vi "Swerve Goto.vi"(1 "Target Angle":dbl, 2 "Target Y":dbl, 3 "Target X":dbl, 4 "Max Speed":dbl) -> (0 "Done":bool)   [LabVIEW 2016, in "Apple script.lvlib"]
uses:
  Apple script.lvlib
  Robot Global Data.vi
  <vilib>/addons/control/pid/NI_PID_pid.lvlib
  <vilib>/addons/control/pid/pid.llb/PID (DBL).vi
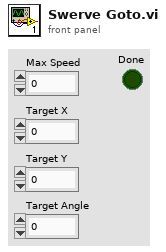
[diagram p1: front panel]
types:
  T1 = enum16{"Prepare to Rotate", "Rotate", "Prepare to Move", "Move", "Done"}
  T2 = cluster{"proportional gain (Kc)":dbl, "integral time (Ti, min)":dbl, "derivative time (Td, min)":dbl}
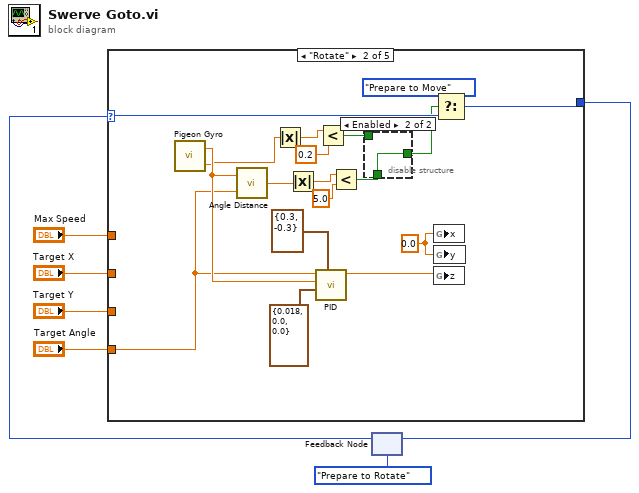
[diagram p0: block diagram]
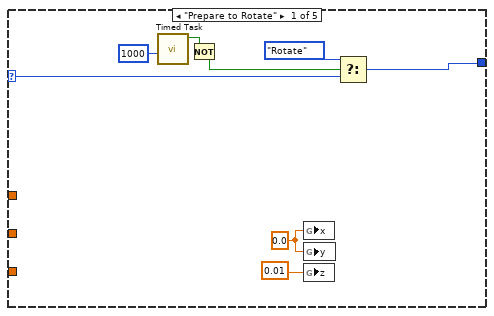
[diagram p2: hidden frame]
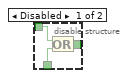
[diagram p3: hidden frame]
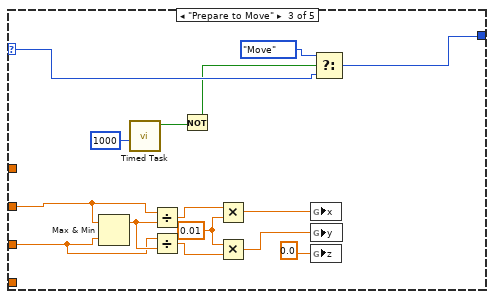
[diagram p4: hidden frame]
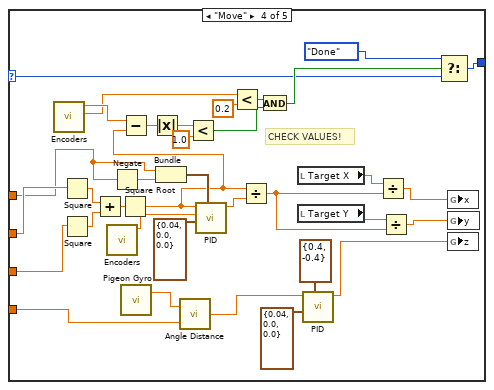
[diagram p5: hidden frame]
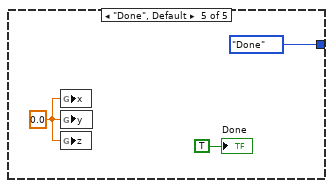
[diagram p6: hidden frame]
diagram:
  n1 = feedback #1(T1."Prepare to Rotate") -> (w6:T1)
  n2 = case shown="\"Rotate\"" w6 {
    selector: w6 -> [w11 w31 w43 w56 _]
    tunnel: [w9 w32 w42 w54 T1."Done"] -> w7
    tunnel: "Max Speed" -> [_ _ _ w59 _]
    tunnel: "Target X" -> [_ _ w45 w60 _]
    tunnel: "Target Y" -> [_ _ w44 w58 _]
    tunnel: "Target Angle" -> [_ w25 _ w57 _]
    frame "Prepare to Rotate" {
      w15 = 0.0
      n3 = call "Timed Task.vi"("Time (ms)"=1000) -> ("Running"=w12:bool)  [unwired: 10 in]
      n4 = Not(x=w12) -> (.not. x?=w8:bool)
      n5 = global write "Robot Global Data.vi" "x"(w15) -> ()
      n6 = global write "Robot Global Data.vi" "y"(w15) -> ()
      n7 = global write "Robot Global Data.vi" "z"(0.01) -> ()
      n8 = Select(t=T1."Rotate", s=w8, f=w11) -> (s? t:f=w9:T1)
    }
    frame "Rotate" {
      w30 = 0.0
      n9 = call "Pigeon Gyro.vi"() -> ("YPR.Yaw"=w26:dbl, "YPR.Yaw Rate"=w20:dbl)  [unwired: 1 in]
      n10 = call "Angle Distance.vi"("target angle"=w25, "current angle"=w26) -> ("distance"=w24:dbl)
      n11 = Absolute Value(x=w20) -> (abs(x)=w21:dbl)
      n12 = Absolute Value(x=w24) -> (abs(x)=w23:dbl)
      n13 = call-poly <vilib>:"PID.vi"("output range"=cluster{"output high":dbl, "output low":dbl} {"output high"=0.3, "output low"=-0.3}, "PID gains"=T2 {"proportional gain (Kc)"=0.018, "integral time (Ti, min)"=0.0, "derivative time (Td, min)"=0.0}, "process variable"=w26, "setpoint"=w25) -> ("output"=w29:dbl)  [unwired: 6 in, 1 out]
      n14 = Less?(x=w21, y=0.2) -> (x < y?=w17:bool)
      n15 = Less?(x=w23, y=5.0) -> (x < y?=w18:bool)
      n16 = disable-structure shown="Enabled" {
        disable-tunnel: w18 -> [w36 w37]
        disable-tunnel: w17 -> [w35 _]
        disable-tunnel: [w34 w37] -> w16
        frame Disabled {
          n17 = Or(x=w35, y=w36) -> (x .or. y?=w34:bool)
        }
        frame Enabled {
        }
      }
      n18 = global write "Robot Global Data.vi" "x"(w30) -> ()
      n19 = global write "Robot Global Data.vi" "y"(w30) -> ()
      n20 = global write "Robot Global Data.vi" "z"(w29) -> ()
      n21 = Select(t=T1."Prepare to Move", s=w16, f=w31) -> (s? t:f=w32:T1)
    }
    frame "Prepare to Move" {
      w51 = 0.01 ("y")
      n22 = Max & Min(x=w45, y=w44) -> (max(x,y)=w52:dbl)  [unwired: 1 out]
      n23 = call "Timed Task.vi"("Time (ms)"=1000) -> ("Running"=w40:bool)  [unwired: 10 in]
      n24 = Divide(x=w45, y=w52) -> (x/y=w49:dbl)
      n25 = Divide(x=w44, y=w52) -> (x/y=w50:dbl)
      n26 = Not(x=w40) -> (.not. x?=w38:bool)
      n27 = Multiply(x=w49, y=w51) -> (x*y=w46:dbl)
      n28 = Multiply(x=w51, y=w50) -> (x*y=w47:dbl)
      n29 = global write "Robot Global Data.vi" "x"(w46) -> ()
      n30 = global write "Robot Global Data.vi" "y"(w47) -> ()
      n31 = global write "Robot Global Data.vi" "z"(0.0 ("Z")) -> ()
      n32 = Select(t=T1."Move", s=w38, f=w43) -> (s? t:f=w42:T1)
    }
    frame "Move" {
      # "CHECK VALUES!"
      n33 = call "Encoders.vi"() -> ("Total Distance"=w65:dbl, "Avg Rate"=w64:dbl)  [unwired: 3 in, 2 out]
      n34 = Square(x=w60) -> (x^2=w86:dbl)
      n35 = Square(x=w58) -> (x^2=w85:dbl)
      n36 = Add(x=w86, y=w85) -> (x+y=w84:dbl)
      n37 = call "Encoders.vi"() -> ("Total Distance"=w66:dbl)  [unwired: 3 in, 3 out]
      n38 = Negate(x=w59) -> (-x=w82:dbl)
      n39 = Square Root(x=w84) -> (sqrt(x)=w71:dbl)
      n40 = Subtract(x=w65, y=w71) -> (x-y=w75:dbl)
      n41 = call "Pigeon Gyro.vi"() -> ("YPR.Yaw"=w67:dbl)  [unwired: 1 in, 1 out]
      n42 = Absolute Value(x=w75) -> (abs(x)=w76:dbl)
      n43 = Bundle("Max Speed"=w59, w82) -> (w83:cluster{"Max Speed":dbl, dbl})  [unwired: 1 in]
      n44 = call "Angle Distance.vi"("target angle"=w57, "current angle"=w67) -> ("distance"=w68:dbl)
      n45 = Less?(x=w76, y=1.0) -> (x < y?=w73:bool)
      n46 = call-poly <vilib>:"PID.vi"("output range"=w83, "PID gains"=T2 {"proportional gain (Kc)"=0.04, "integral time (Ti, min)"=0.0, "derivative time (Td, min)"=0.0}, "process variable"=w66, "setpoint"=w71) -> ("output"=w79:dbl)  [unwired: 6 in, 1 out]
      n47 = Less?(x=w64, y=0.2) -> (x < y?=w74:bool)
      n48 = Divide(x=w71, y=w79) -> (x/y=w80:dbl)
      n49 = And(x=w74, y=w73) -> (x .and. y?=w72:bool)
      n50 = local read "Target X"() -> (w55:dbl)
      n51 = local read "Target Y"() -> (w81:dbl)
      n52 = call-poly <vilib>:"PID.vi"("output range"=cluster{"output high":dbl, "output low":dbl} {"output high"=0.4, "output low"=-0.4}, "PID gains"=T2 {"proportional gain (Kc)"=0.04, "integral time (Ti, min)"=0.0, "derivative time (Td, min)"=0.0}, "setpoint"=w68) -> ("output"=w61:dbl)  [unwired: 7 in, 1 out]
      n53 = Divide(x=w55, y=w80) -> (x/y=w63:dbl)
      n54 = Divide(x=w81, y=w80) -> (x/y=w62:dbl)
      n55 = Select(t=T1."Done", s=w72, f=w56) -> (s? t:f=w54:T1)
      n56 = global write "Robot Global Data.vi" "x"(w63) -> ()
      n57 = global write "Robot Global Data.vi" "y"(w62) -> ()
      n58 = global write "Robot Global Data.vi" "z"(w61) -> ()
    }
    frame "Done", Default {
      w90 = 0.0
      n59 = global write "Robot Global Data.vi" "x"(w90) -> ()
      n60 = global write "Robot Global Data.vi" "y"(w90) -> ()
      n61 = global write "Robot Global Data.vi" "z"(w90) -> ()
      "Done" <- TRUE ("Done")
    }
  }
  n62 = feedback-in #1(w7) -> ()
